vi "Initialize Outputs.vi"(8 "error in":errorcluster, 11 "PIOD in":refnum<class "PIOD.lvclass">) -> (0 "error out":errorcluster, 3 "PIOD out":refnum<class "PIOD.lvclass">)   [LabVIEW 2018, in "PIOD.lvlib" / "PIOD.lvclass"]
uses:
  PIOD.lvclass
  builds/Configuration.lvlibp/Configuration.lvclass
  builds/PLC.lvlibp/PLC.lvclass
  C:/Users/Ron.Dexter.LUMINARTECH/Desktop/builds/PLC.lvlibp/PLC.lvclass
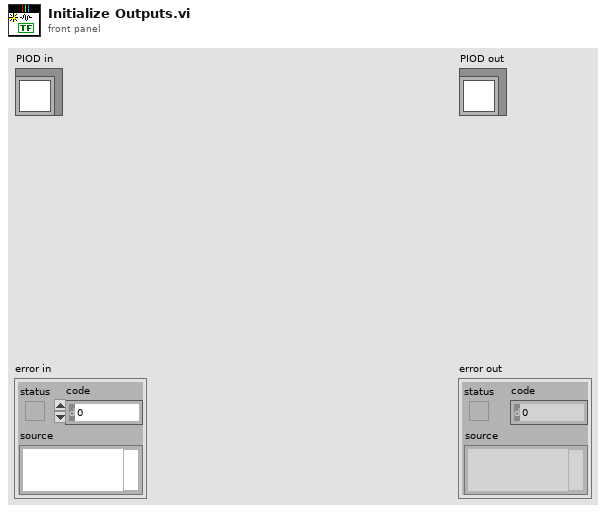
[diagram p1: front panel]
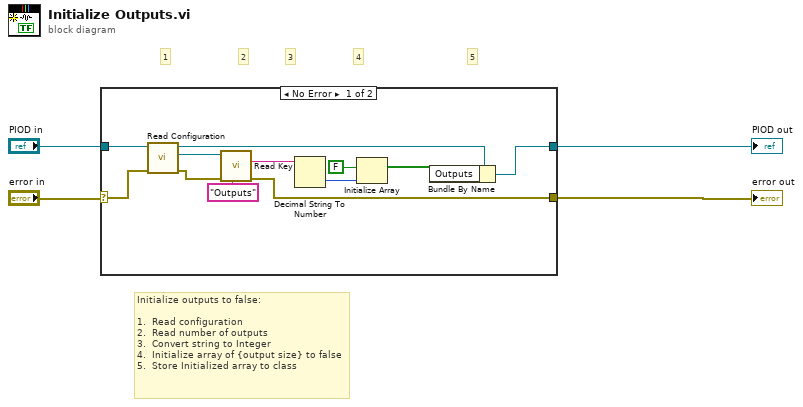
[diagram p0: block diagram]
diagram:
  # "Initialize outputs to false:\n\n1.  Read configuration\n2.  Read number of outputs\n3.  Convert string to Integer\n4.  Initialize array of {output size} to false\n5.  Store Initialized array to class"
  # "5"
  # "4"
  # "3"
  # "2"
  # "1"
  n1 = case shown="No Error" "error in" {
    selector: "error in" -> [w15 w18]
    tunnel: [w5 w18] -> w2
    tunnel: [w6 w17] -> w1
    tunnel: "PIOD in" -> [w16 w17]
    frame No Error {
      n2 = call "Read Configuration.vi"("error in (no error)"=w15, "PLC in"=w16) -> ("error out"=w13:errorcluster, "Configuration"=w14:refnum<class "Configuration.lvclass">, "PLC out"=w8:refnum<class "PIOD.lvclass">)  [unwired: 7 in]
      n3 = call "Read Key.vi"("Key:"="Outputs", "error in"=w13, "Configuration in"=w14) -> ("error out"=w5:errorcluster, "Value"=w11:string)  [unwired: 6 in, 1 out]
      n4 = Decimal String To Number(string=w11) -> (number=w10:i32)  [unwired: 2 in, 1 out]
      n5 = Initialize Array(FALSE, w10) -> (w7:bool[])
      n6 = Bundle By Name(cluster=w8, "Outputs"=w7) -> (w6:refnum<class "PIOD.lvclass">)
    }
    frame Error {
    }
  }
  "error out" <- w2
  "PIOD out" <- w1
